vi "TD_Create_File_Single.vi"(7 "Parent Folder ID (optional)":string, 8 "error in (no error)":errorcluster, 10 "File name":string="labviewFile", 11 "TekDrive Session":T3) -> (0 "error out":errorcluster, 2 "value":T2, 3 "TekDrive Session 2":T3, 4 "body":string, 5 "headers":string)   [LabVIEW 2018]
uses:
  Controls/TekDriveSession.ctl
  <vilib>/httpClient/ClientHandle.ctl
  Controls/File Model.ctl
  <vilib>/httpClient/POSTBuffer.vi
  <vilib>/httpClient/LabVIEWHTTPClient.lvlib
panel:
  # "{\n    \"name\": \"my_new_file.txt\",\n    \"parentFolderId\": \"ec054c96-f120-480a-a3a0-c984024e946e\"\n}"
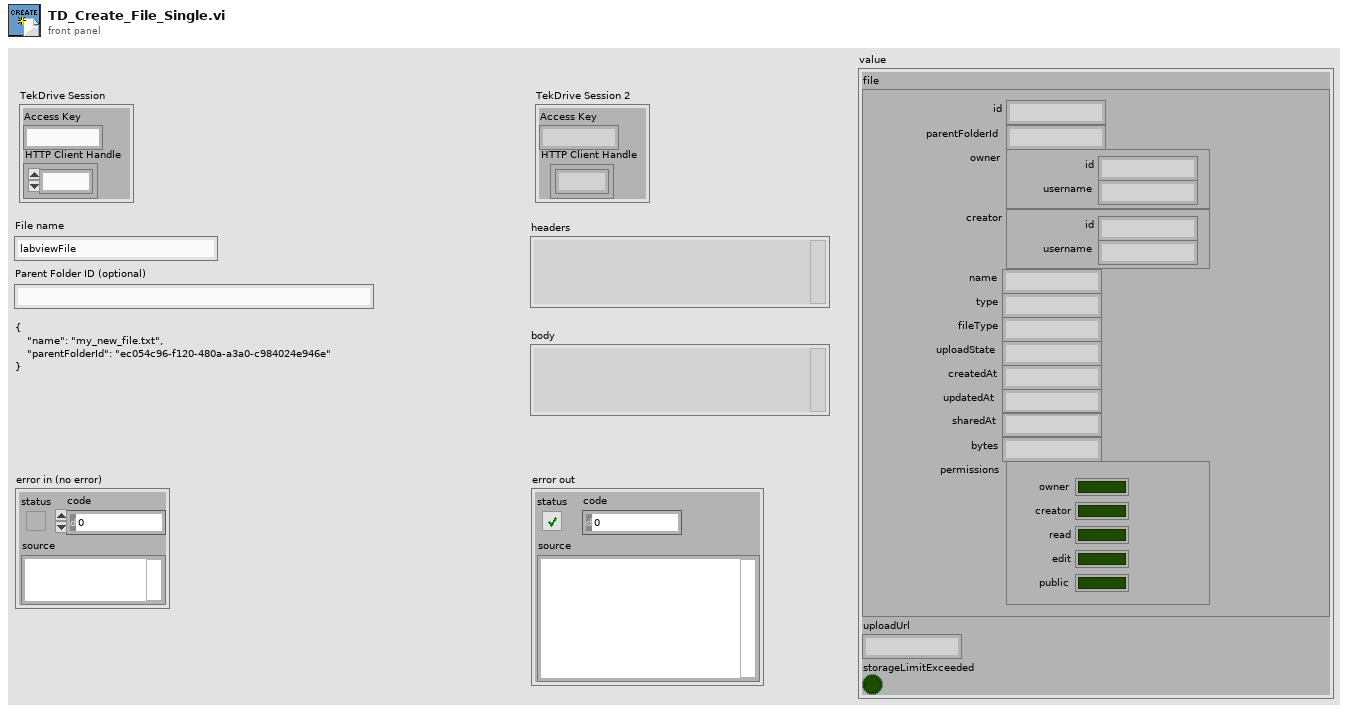
[diagram p1: front panel]
types:
  T1 = typedef "File Model.ctl" = cluster{"id":string, "parentFolderId":string, "owner":cluster{"id":string, "username":string}, "creator":cluster{"id":string, "username":string}, "name":string, "type":string, "fileType":string, "uploadState":string, "createdAt":string, "updatedAt":string, "sharedAt":string, "bytes":string, "permissions":cluster{"owner":bool, "creator":bool, "read":bool, "edit":bool, "public":bool}}
  T2 = cluster{"file":T1, "uploadUrl":string, "storageLimitExceeded":bool}
  T3 = typedef "TekDriveSession.ctl" = cluster{"Access Key":string, "HTTP Client Handle":T4}
  T4 = typedef "LabVIEWHTTPClient.lvlib/ClientHandle.ctl" = refnum<k1>
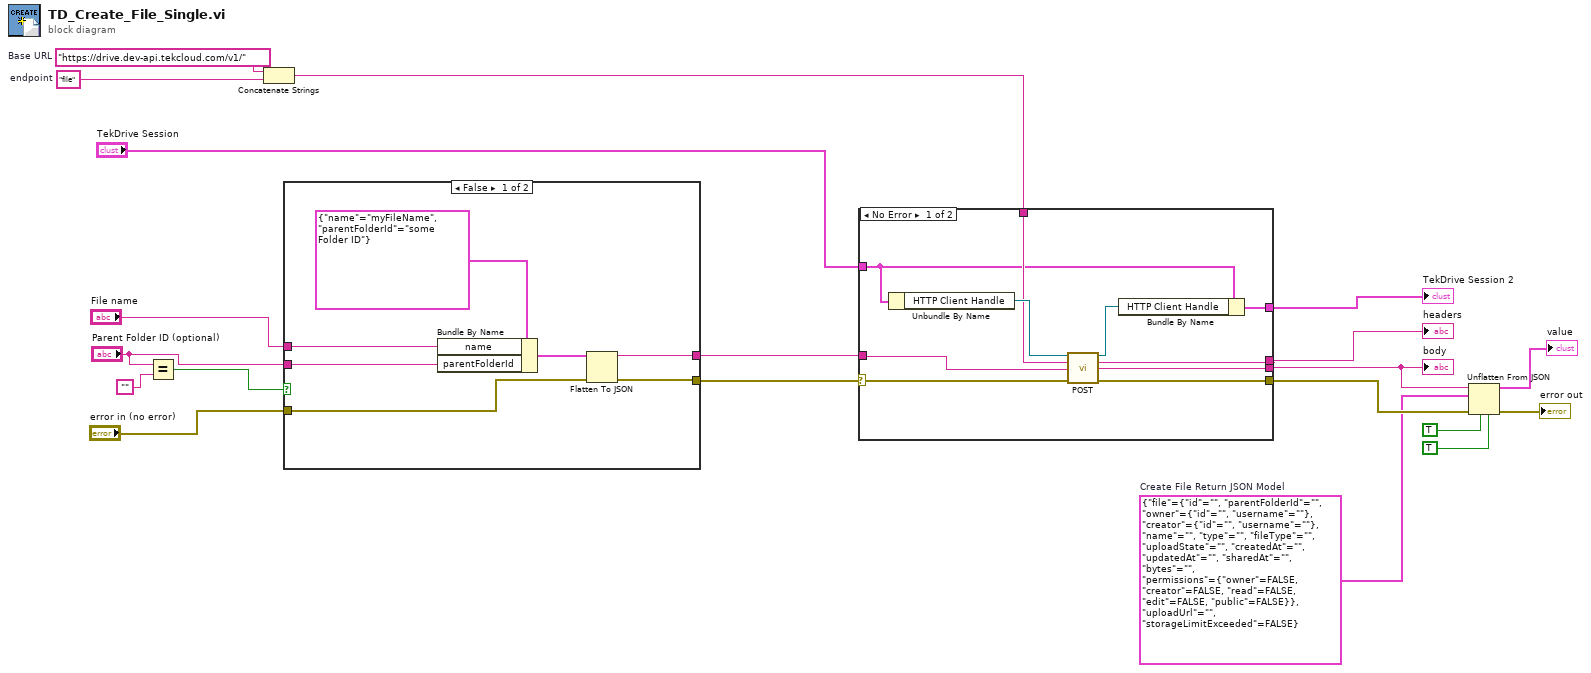
[diagram p0: block diagram]
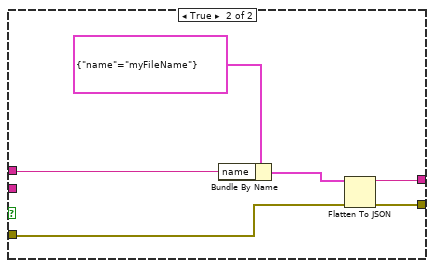
[diagram p2: hidden frame]
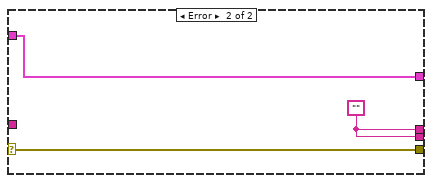
[diagram p3: hidden frame]
diagram:
  w4 = T2 {"file"={"id"="", "parentFolderId"="", "owner"={"id"="", "username"=""}, "creator"={"id"="", "username"=""}, "name"="", "type"="", "fileType"="", "uploadState"="", "createdAt"="", "updatedAt"="", "sharedAt"="", "bytes"="", "permissions"={"owner"=FALSE, "creator"=FALSE, "read"=FALSE, "edit"=FALSE, "public"=FALSE}}, "uploadUrl"="", "storageLimitExceeded"=FALSE}  # Create File Return JSON Model
  w18 = "file"  # endpoint
  w19 = "https://drive.dev-api.tekcloud.com/v1/"  # Base URL
  n1 = Equal?(x="Parent Folder ID (optional)", y="") -> (x = y?=w11:bool)
  n2 = Concatenate Strings(w19, w18) -> (w17:string)
  n3 = case shown="False" w11 {
    tunnel: [w22 w29] -> w14
    tunnel: "error in (no error)" -> [w25 w30]
    tunnel: "Parent Folder ID (optional)" -> [w24 _]
    tunnel: "File name" -> [w23 w31]
    tunnel: [w21 w28] -> w8
    frame False {
      n4 = Bundle By Name(cluster=cluster{"name":string, "parentFolderId":string} {"name"="myFileName", "parentFolderId"="some Folder ID"}, "name"=w23, "parentFolderId"=w24) -> (w26:cluster{"name":string, "parentFolderId":string})
      n5 = Flatten To JSON(anything=w26, error in (no error)=w25) -> (JSON string=w22:string, 11:w21:errorcluster)  [unwired: 1 in]
    }
    frame True {
      n6 = Bundle By Name(cluster=cluster{"name":string} {"name"="myFileName"}, "name"=w31) -> (w33:cluster{"name":string})
      n7 = Flatten To JSON(anything=w33, error in (no error)=w30) -> (JSON string=w29:string, 11:w28:errorcluster)  [unwired: 1 in]
    }
  }
  n8 = case shown="No Error" w8 {
    selector: w8 -> [w34 w45]
    tunnel: "TekDrive Session" -> [w41 w46]
    tunnel: w17 -> [w42 _]
    tunnel: w14 -> [w35 _]
    tunnel: [w39 w45] -> w6
    tunnel: [w38 w44] -> w7
    tunnel: [w37 w44] -> w16
    tunnel: [w36 w46] -> w15
    frame No Error {
      n9 = Unbundle By Name(w41) -> ("HTTP Client Handle"=w43:T4)
      n10 = call-poly <vilib>:"POST.vi"("client handle"=w43, "url"=w42, "buffer"=w35, "error in (no error)"=w34) -> ("client handle out"=w40:T4, "headers"=w37:string, "body"=w38:string, "error out"=w39:errorcluster)  [unwired: 8 in]
      n11 = Bundle By Name(cluster=w41, "HTTP Client Handle"=w40) -> (w36:T3)
    }
    frame Error {
      w44 = ""
    }
  }
  "body" <- w7
  "headers" <- w16
  "TekDrive Session 2" <- w15
  n12 = Unflatten From JSON(JSON string=w7, type and defaults=w4, default null elements? (F)=TRUE, strict validation? (F)=TRUE, error in (no error)=w6) -> (value=→"value":T2, error out=→"error out":errorcluster)  [unwired: 2 in]
